vi "gfitsio-get-hdu-list.vi"(8 "error in (no error)":errorcluster, 11 "gfits refnum":T2) -> (0 "error out":errorcluster, 1 "hdu types":T1[](array[typedef]) items=["ANY_HDU"=-1, "IMAGE_HDU"=0, "ASCII_TBL"=1, "BINARY_TBL"=2], 2 "hdu names":string[](array[string]), 3 "dup gfits refnum":T2)   [LabVIEW 2019, in "gfitsio.lvlib"]
doc: "Return a list of HDUs in the FITS file. The list is returned in two 1D arrays: \n\nAn array of strings contains the names (if they are stored in the EXTNAME keyword) of each HDU. If the HDU is unnamed the corresponding string will be empty.\n\nAn array of enumerations contains the type of each HDU (image, binary table or ascii table)."
uses:
  gfitsio.lvlib
  gfitsio-refnum.ctl
  cfitsio-hdutypes.ctl
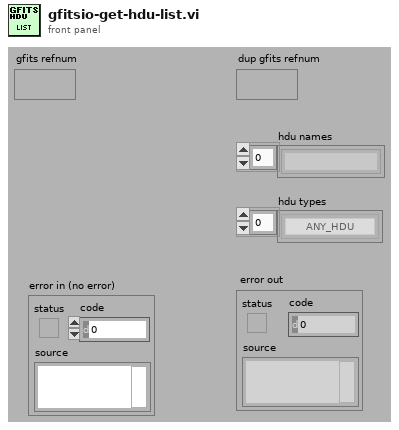
[diagram p1: front panel]
types:
  T1 = typedef "gfitsio.lvlib/cfitsio-hdutypes.ctl" = i32
  T2 = typedef "gfitsio.lvlib/gfitsio-refnum.ctl" = refnum<k1>
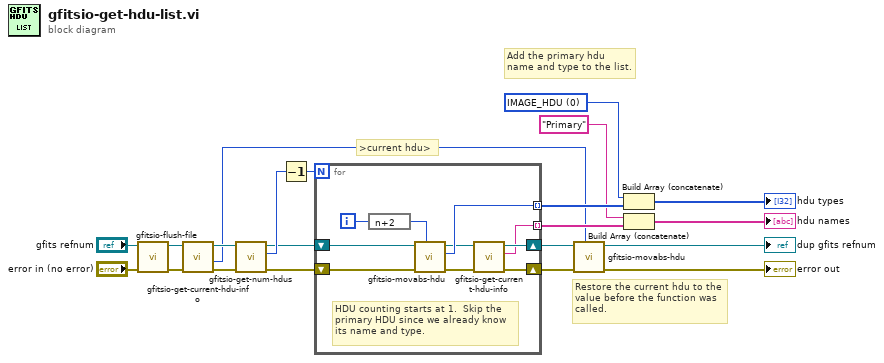
[diagram p0: block diagram]
diagram:
  w6 = T1 0 items=["ANY_HDU"=-1, "IMAGE_HDU"=0, "ASCII_TBL"=1, "BINARY_TBL"=2] ("hdutype")
  # ">current hdu>"
  # "Restore the current hdu to the value before the function was called."
  # "Add the primary hdu name and type to the list."
  n1 = call "gfitsio-flush-file.vi"("error in (no error)"="error in (no error)", "gfits refnum"="gfits refnum") -> ("error out"=w4:errorcluster, "dup gfits refnum"=w3:T2)  [unwired: 8 out]
  n2 = call "gfitsio-get-current-hdu-info.vi"("error in (no error)"=w4, "gfits refnum"=w3) -> ("error out"=w16:errorcluster, "hdu number"=w5:i32, "dup gfits refnum"=w15:T2)  [unwired: 7 out]
  n3 = call "gfitsio-get-num-hdus.vi"("error in (no error)"=w16, "gfits refnum"=w15) -> ("error out"=w8:errorcluster, "number of hdus"=w21:i32, "dup gfits refnum"=w7:T2)  [unwired: 7 out]
  n4 = Decrement(x=w21) -> (x-1=w20:i32)
  n5 = for {
    N: w20 -> [_]
    shift-right: [w23] -> w14
    shift-left: w8 -> [w31]
    shift-right: [w25] -> w13
    shift-left: w7 -> [w30]
    tunnel: [w28] -> w19 mode=indexing
    tunnel: [w24] -> w18 mode=indexing
    i -> [w29]
    # "HDU counting starts at 1.  Skip the primary HDU since we already know its name and type."
    n6 = expression code="n+2"(w29) -> (w22:i32)
    n7 = call "gfitsio-movabs-hdu.vi"("hdunum"=w22, "error in (no error)"=w31, "gfits refnum"=w30) -> ("error out"=w27:errorcluster, "hdutype"=w28:T1, "dup gfits refnum"=w26:T2)  [unwired: 2 in, 4 out]
    n8 = call "gfitsio-get-current-hdu-info.vi"("error in (no error)"=w27, "gfits refnum"=w26) -> ("error out"=w23:errorcluster, "hdu name"=w24:string, "dup gfits refnum"=w25:T2)  [unwired: 7 out]
  }
  n9 = call "gfitsio-movabs-hdu.vi"("hdunum"=w5, "error in (no error)"=w14, "gfits refnum"=w13) -> ("error out"=→"error out":errorcluster, "dup gfits refnum"=→"dup gfits refnum":T2)  [unwired: 2 in, 5 out]
  n10 = Build Array (concatenate)(w6, w19) -> (→"hdu types":T1[])
  n11 = Build Array (concatenate)("Primary" ("keyname"), w18) -> (→"hdu names":string[])
